vi "Y Goal Marker.vi"(6 "goal x":dbl, 7 "Touch":bool, 9 "y":dbl, 10 "x":dbl, 11 "dest_y_kick":dbl) -> (2 "kick error":dbl)   [LabVIEW 2016]
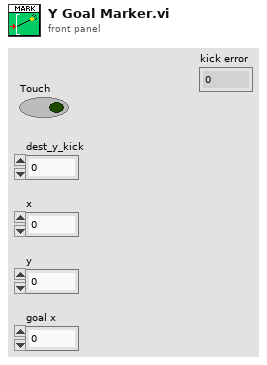
[diagram p1: front panel]
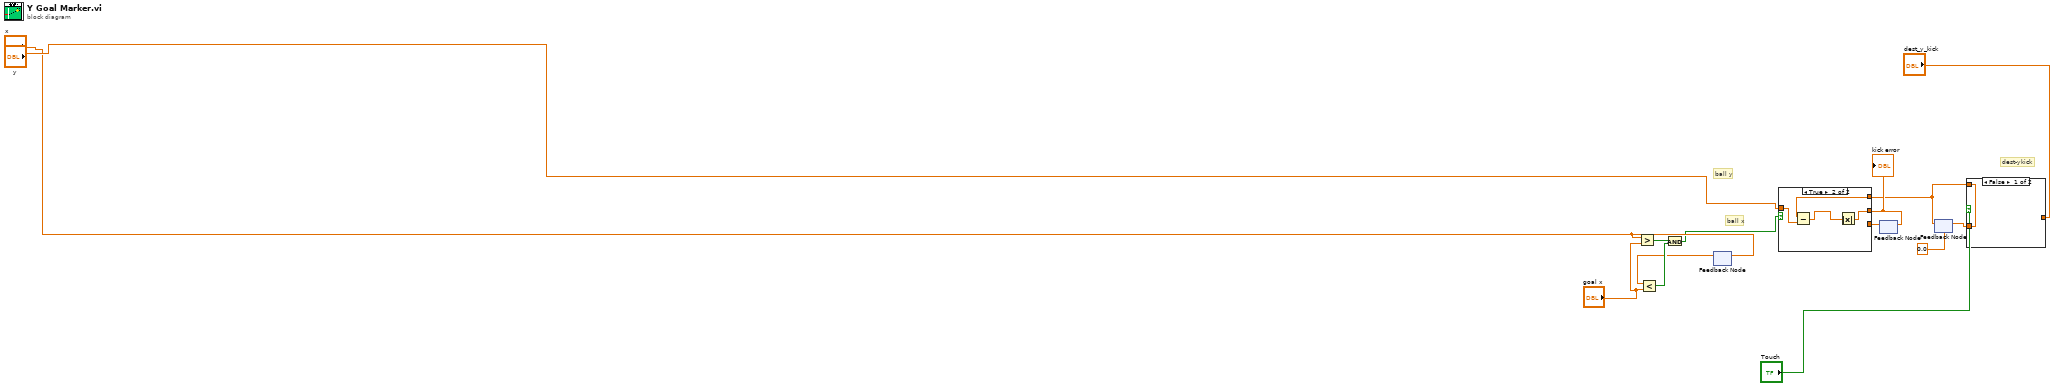
[diagram p0: block diagram]
diagram:
  # "dest-ykick"
  # "ball y"
  # "ball x"
  n1 = Greater?(x="x", y="goal x") -> (0:w6:bool)
  n2 = feedback #1() -> (w5:dbl)  [unwired: 1 in]
  n3 = Less?(x=w5, y="goal x") -> (x < y?=w7:bool)
  n4 = And(x=w6, y=w7) -> (x .and. y?=w9:bool)
  n5 = feedback-in #1("x") -> ()
  n6 = feedback #2() -> (w13:dbl)  [unwired: 1 in]
  n7 = feedback #3(0.0 ("dest_y")) -> (w10:dbl)
  n8 = case shown="True" w9 {
    tunnel: w10 -> [_ w19]
    tunnel: "y" -> [_ w16]
    tunnel: [w15 w17] -> w12
    tunnel: w13 -> [w15 _]
    frame False {
    }
    frame True {
      n9 = Subtract(x=w19, y=w16) -> (x-y=w18:dbl)
      n10 = Absolute Value(x=w18) -> (abs(x)=w17:dbl)
    }
  }
  "kick error" <- w12
  n11 = feedback-in #2(w12) -> ()
  n12 = case shown="False" "Touch" {
    tunnel: "dest_y_kick" -> [_ w21]
    tunnel: [w20 w21] -> w3
    tunnel: w10 -> [w20 _]
    frame False {
    }
    frame True {
    }
  }
  n13 = feedback-in #3(w3) -> ()
